vi "DecimalPlace.vi"(6 "Dp":i8, 10 "Input":dbl=0.125464827 format="%#_13g") -> (3 "Output":dbl)   [LabVIEW 2014]
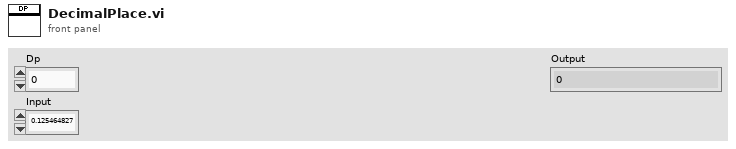
[diagram p1: front panel]
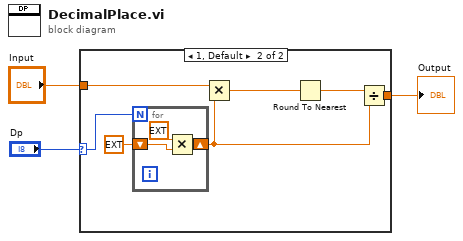
[diagram p0: block diagram]
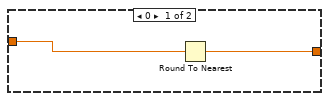
[diagram p2: hidden frame]
diagram:
  n1 = case shown="1, Default" "Dp" {
    selector: "Dp" -> [_ w6]
    tunnel: "Input" -> [w4 w9]
    tunnel: [w5 w10] -> w2
    frame 0 {
      n2 = Round To Nearest(number=w4) -> (nearest integer value=w5:dbl)
    }
    frame 1, Default {
      n3 = for {
        N: w6 -> [_]
        shift-right: [w14] -> w8
        shift-left: ext 10.0 ("x") -> [w13]
        n4 = Multiply(x=ext 10.0, y=w13) -> (x*y=w14:ext)
      }
      n5 = Multiply(x=w9, y=w8) -> (x*y=w12:ext)
      n6 = Round To Nearest(number=w12) -> (nearest integer value=w11:ext)
      n7 = Divide(x=w11, y=w8) -> (x/y=w10:ext)
    }
  }
  "Output" <- w2
